vi "Write_comp_data.vi"(3 "error in":errorcluster, 4 "comp_data":T1(array[cluster]), 5 "ref in":i32) -> (0 "error out":errorcluster, 2 "ref out":i32)   [LabVIEW 2010]
uses:
  <vilib>/addons/h5labview2/dataset/H5Dwrite.llb/H5Dwrite.xnode
  <vilib>/addons/h5labview2/base/H5Equery.vi
  <vilib>/addons/h5labview2/group/H5G.lvlib
  <vilib>/addons/h5labview2/h5labview.lib
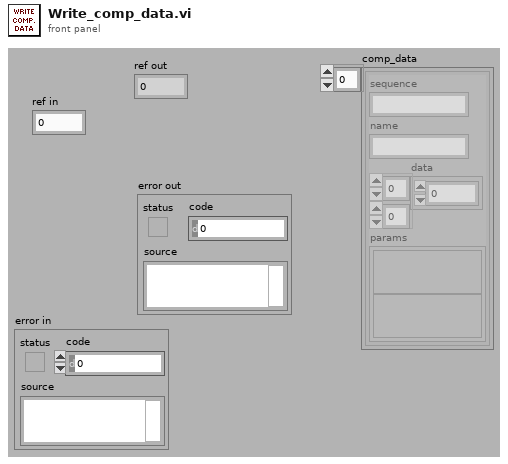
[diagram p1: front panel]
types:
  T1 = cluster{"sequence":string, "name":string, "data":sgl[][], "params":variant[]}[]
  T2 = typedef "hid_t.ctl" = i32
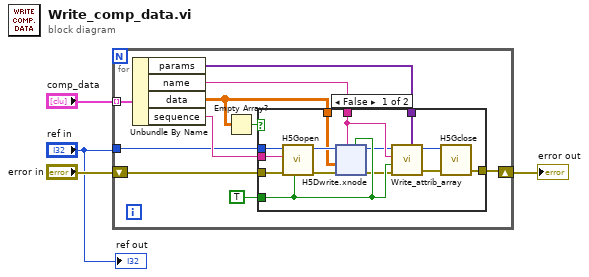
[diagram p0: block diagram]
diagram:
  n1 = for {
    tunnel: "comp_data" -> [w13] mode=indexing
    shift-right: [w8] -> w4
    shift-left: "error in" -> [w14]
    tunnel: "ref in" -> [w11]
    n2 = Unbundle By Name(w13) -> ("params"=w10:variant[], "name"=w9:string, "data"=w6:sgl[][], "sequence"=w12:string)
    n3 = Empty Array?(array=w6) -> (empty?=w5:bool)
    n4 = case shown="False" w5 {
      tunnel: w14 -> [w25 w46]
      tunnel: w12 -> [w26 _]
      tunnel: w11 -> [w27 _]
      tunnel: w10 -> [w28 _]
      tunnel: w9 -> [w23 _]
      tunnel: [w19 w46] -> w8
      tunnel: TRUE ("Create if not found (F)") -> [w20 _]
      tunnel: w6 -> [w21 _]
      frame False {
        n5 = call <vilib>:"H5Gopen.vi"("create? (F)"=w20, "error in (no error)"=w25, "name"=w26, "ref in"=w27) -> ("error out"=w22:errorcluster, "group out"=w24:T2)  [unwired: 3 in]
        n6 = xnode "H5Dwrite.xnode"("replace? (F)"=w20, "dataset name"=w23, "error in (no error)"=w22, "data"=w21, "ref in"=w24) -> ("error out"=w15:errorcluster, "ref out"=w16:i32)  [unwired: 2 in, 1 out]
        n7 = call <userlib>:"Write_attrib_array.vi"("attribs"=w28, "error in (no error)"=w15, "overwrite?"=w20, "obj_name"=w23, "ref"=w16) -> ("error out"=w18:errorcluster, "ref out"=w17:i32)  [unwired: 3 in]
        n8 = call <vilib>:"H5Gclose.vi"("error in (no error)"=w18, "group in"=w17) -> ("error out"=w19:errorcluster)  [unwired: 3 in]
      }
      frame True {
      }
    }
  }
  "error out" <- w4
  "ref out" <- "ref in"
